vi "Start Measurement.vi"(8 "error in":errorcluster, 9 "pin map context":T3, 10 "measurement configuration":T1={"double array in"=[3.4, 5.6], "double in"=1.2, "U32 array in"=[32, 33], "U32 in"=32, "U64 array in"=[64, 65], "U64 in"=64, "I32 array in"=[-32, -33], "I32 in"=-32, "I64 array in"=[-64, -65], "I64 in"=-64, "bool in"=TRUE, "string in"="Lorem ipsum dolor sit", "u32 color ring in"=1, "u32 animal enum in"=enum."Gopher"}, 11 "gRPCid in":T2) -> (0 "error out":errorcluster, 2 "call id":T2, 3 "gRPCid out":T2)   [LabVIEW 2025, in "Automotive-Ethernet_LabVIEW.lvlib"]
doc: "Start the measurement for the given measurement configuration."
uses:
  Automotive-Ethernet_LabVIEW.lvlib
  <vilib>/gRPC/Generated APIs/ni/measurementlink/measurement/v2/Measurement Service Client V2/RPC Messages/ni_measurementlink_PinMapContext.ctl
  <vilib>/gRPC/LabVIEW gRPC Library/Shared/grpcId.ctl
  controls/Measurement Configuration.ctl
  <vilib>/gRPC/Generated APIs/ni/measurementlink/measurement/v2/Measurement Service Client V2/RPC Messages/ni_measurementlink_measurement_v2_MeasureRequest.ctl
  <vilib>/gRPC/Generated APIs/ni/measurementlink/measurement/v2/Measurement Service Client V2/RPC Messages/google_protobuf_Any.ctl
  7061fa50-9f43-4eb3-8fe8-31484f53e761.vi
  <vilib>/gRPC/LabVIEW gRPC Library/Server API/Translate Protobuf Error.vi
  <vilib>/AdvancedString/1D String Array to Delimited String.vi
  <vilib>/gRPC/LabVIEW gRPC Library/Server API/Server/Get Server DLL Path.vi
  <vilib>/gRPC/Generated APIs/ni/measurementlink/measurement/v2/Measurement Service Client V2/Measurement Service Client V2.lvlib
  <vilib>/gRPC/LabVIEW gRPC Library/grpc-lvsupport-release.lvlib
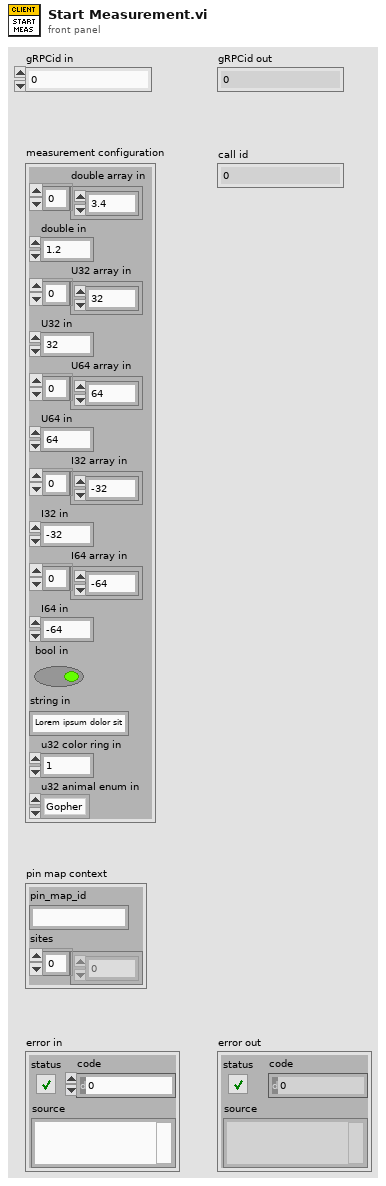
[diagram p1: front panel]
types:
  T1 = typedef "Automotive-Ethernet_LabVIEW.lvlib/Measurement Configuration.ctl" = cluster{"double array in":dbl[], "double in":dbl, "U32 array in":u32[], "U32 in":u32, "U64 array in":u64[], "U64 in":u64, "I32 array in":i32[], "I32 in":i32, "I64 array in":i64[], "I64 in":i64, "bool in":bool, "string in":string, "u32 color ring in":u32, "u32 animal enum in":enum32{"Rabbit", "Gopher", "Badger"}}
  T2 = typedef "grpc-lvsupport-release.lvlib/grpcId.ctl" = u64
  T3 = typedef "Measurement Service Client V2.lvlib/ni_measurementlink_PinMapContext.ctl" = cluster{"pin_map_id":string, "sites":i32[]}
  T4 = typedef "Measurement Service Client V2.lvlib/ni_measurementlink_measurement_v2_MeasureRequest.ctl" = cluster{"configuration_parameters":T5, "pin_map_context":T3}
  T5 = typedef "Measurement Service Client V2.lvlib/google_protobuf_Any.ctl" = cluster{"type_url":string, "value":u8[]}
  T6 = typedef "grpc-lvsupport-release.lvlib/Any.ctl" = cluster{"Type Url":string, "Bytes":u8[]}
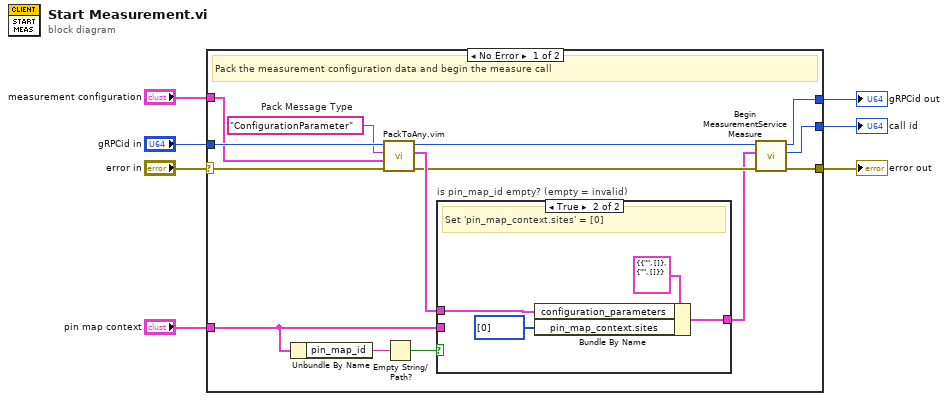
[diagram p0: block diagram]
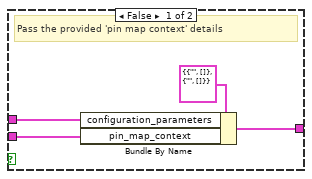
[diagram p2: hidden frame]
diagram:
  n1 = case shown="No Error" "error in" {
    selector: "error in" -> [w18 w30]
    tunnel: "pin map context" -> [w21 _]
    tunnel: "gRPCid in" -> [w19 _]
    tunnel: [w15 w30] -> w4
    tunnel: [w14 _] -> w3
    tunnel: [w13 _] -> w2
    tunnel: "measurement configuration" -> [w10 _]
    frame No Error {
      w11 = "ConfigurationParameter"  # Pack Message Type
      # "Pack the measurement configuration data and begin the measure call"
      n2 = Unbundle By Name(w21) -> ("pin_map_id"=w9:string)
      n3 = call "PackToAny.vim"("error in"=w18, "Data To Pack"=w10, "Message Type"=w11, "gRPCid in"=w19) -> ("error out"=w17:errorcluster, "Any"=w20:T6, "gRPCid out"=w12:u64)  [unwired: 5 in]
      n4 = Empty String/Path?(string/path=w9) -> (empty?=w8:bool)
      n5 = case "is pin_map_id empty? (empty = invalid)" shown="True" w8 {
        tunnel: [w25 w29] -> w16
        tunnel: w21 -> [w23 _]
        tunnel: w20 -> [w22 w28]
        frame False {
          # "Pass the provided 'pin map context' details"
          n6 = Bundle By Name(cluster=T4 {"configuration_parameters"={"type_url"="", "value"=[]}, "pin_map_context"={"pin_map_id"="", "sites"=[]}} ("Request Data"), "configuration_parameters"=w22, "pin_map_context"=w23) -> (w25:T4)
        }
        frame True {
          # "Set 'pin_map_context.sites' = [0]"
          n7 = Bundle By Name(cluster=T4 {"configuration_parameters"={"type_url"="", "value"=[]}, "pin_map_context"={"pin_map_id"="", "sites"=[]}} ("Request Data"), "configuration_parameters"=w28, "pin_map_context.sites"=i32[] [0]) -> (w29:T4)
        }
      }
      n8 = call <vilib>:"Begin MeasurementService Measure.vi"("error in"=w17, "Request Data"=w16, "gRPC ID"=w12) -> ("error out"=w15:errorcluster, "Call Id Out"=w14:T2, "gRPC ID out"=w13:T2)  [unwired: 6 in]
    }
    frame Error {
      # "Pass"
    }
  }
  "error out" <- w4
  "call id" <- w3
  "gRPCid out" <- w2
